vi "LVCAM Msg Receive.vi"(11 "Process in":refnum<class "Process.lvclass">) -> (0 "error out":errorcluster, 1 "DeQ Msg?":bool, 2 "Msg":refnum<class "Msg.lvclass">, 3 "Process out":refnum<class "Process.lvclass">)   [LabVIEW 2021, in "Process.lvlib" / "Process.lvclass"]
uses:
  Process.lvclass
  LVCAM/LVCAM/Msg/Msg.lvclass
  Process.lvclass/Process.ctl
  LVCAM/LVCAM/LVCAM/LVCAM.lvclass
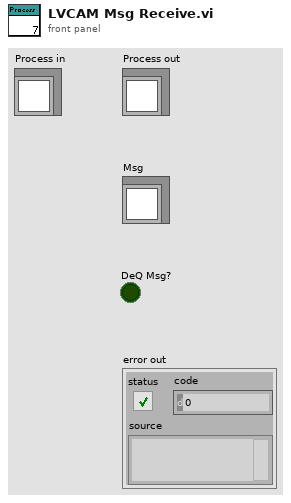
[diagram p1: front panel]
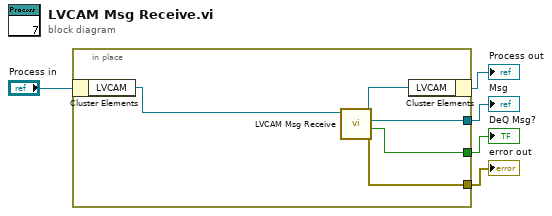
[diagram p0: block diagram]
diagram:
  n1 = in-place {
    in-place-border: [w9] -> w5
    in-place-border: [w8] -> w4
    in-place-border: [w7] -> w3
    n2 = in-place-cluster #1("Process in") -> ("LVCAM"=w6:refnum<class "LVCAM.lvclass">)
    n3 = call-dynamic "LVCAM Msg Receive.vi"("LVCAM Msg Receive in"=w6) -> ("error out"=w7:errorcluster, "DeQ Msg?"=w8:bool, "Msg"=w9:refnum<class "Msg.lvclass">, "LVCAM Msg Receive out"=w10:refnum<class "LVCAM.lvclass">)  [unwired: 7 in]
    n4 = in-place-cluster #1("LVCAM"=w10) -> (→"Process out":refnum<class "Process.lvclass">)
  }
  "DeQ Msg?" <- w4
  "Msg" <- w5
  "error out" <- w3
